vi "Channel Fault - Single.vi"() -> ()   [LabVIEW 2010]
doc: "NI VeriStand custom UI element to fault a single channel. Right-Click on the UI icon to bring up the channel selection dialog and choose a channel. The Path and current value will be displayed.\n\nIn order to fault a channel, set the 'Fault Value' and click the 'Fault Channel?' button. To clear the fault for that channel, click the 'Fault Channel?' button again (so it is false / off)"
uses:
  <vilib>/NI VeriStand/Display Template Support/Display Template Support.llb/cluster_Screen Item Settings.ctl
  <vilib>/NI VeriStand/Display Template Support/Display Template Support.llb/cluster_Graph Scale Settings.ctl
  <vilib>/NI VeriStand/Display Template Support/Display Template Support.llb/cluster_Graph Plot Settings.ctl
  NationalInstruments.VeriStand.SystemStorage
  <vilib>/NI VeriStand/Display Template Support/Display Template Support.llb/enum_Display Template Handler Minimal To Widget Msg.ctl
  <vilib>/NI VeriStand/Display Template Support/Display Template Support.llb/enum_Display Template Handler Minimal To Workspace.ctl
  Data Typedef.ctl
  <vilib>/NI VeriStand/Display Template Support/Display Template Support.llb/sub_Display Template Handler Custom.vi
  <vilib>/NI VeriStand/Execution/Workspace/NI VeriStand - Get Single Channel Value.vi
  <vilib>/NI Veristand/Execution/Workspace/NI_VS Workspace ExecutionAPI.lvlib
  <vilib>/NI Veristand/Execution/ChannelFaultManager/NI_VS ChannelFault ExecutionAPI.lvlib
panel:
  in  "NIVS.System Definition Root":refnum<k24>
  in  "NIVS.Gateway IP Address":string
  out "Fault Channel Full Path":string
  in  "Fault Channel?":bool
  out "Current Value":dbl
  in  "Fault Value":dbl
  in  "Item.Data":T1
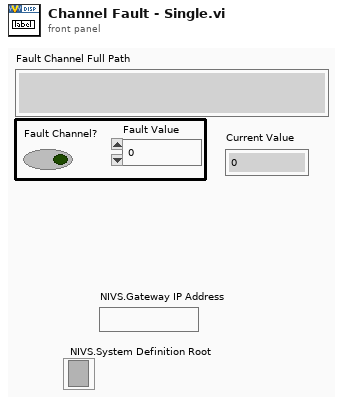
[diagram p1: front panel]
types:
  T1 = typedef "cluster_Screen Item Settings.ctl" = cluster{"Template VI":string, "Position X":i32, "Position Y":i32, "Custom":string, "Show Title Bar":bool, "ID":i32, "Always On Top":bool, "Allow Resize":bool, "Allow Minimize":bool, "Allow Close":bool, "Size to Screen":bool, "Screen.ID":i32, "State":enum16{"Normal", "New"}, "Title":string, "Window Bounds":cluster{"[0]":i16, "[1]":i16, "[2]":i16, "[3]":i16}, "Channel Ref":u64, "Unit":string, "Default Units?":bool, "Flash Limit?":bool, "Color 1":u32, "Color 2":u32, "Color 3":u32, "Color 4":u32, "Bck Color":u32, "Fore Color":u32, "Limit 1":dbl, "Limit 2":dbl, "Limit 3":dbl, "Limit 4":dbl, "Limit Mode 1":i32, "Limit Mode 2":i32, "Limit Mode 3":i32, "Limit Mode 4":i32, "Scale Precision":i32, "Scale Min":dbl, "Scale Max":dbl, "Format":i32, "Precision":i32, "Background Type":i32, "IDs":i32[], "Units":string[], "Labels":string[], "Scale Factor":dbl, "Scale Offset":dbl, "YScale Index":u32[], "XScale":T2, "YScales":T2[], "Plots":T3[], "Update Period":dbl, "History Length":dbl, "My.Ref":refnum<vi>, "Is Control?":bool, "Channel Paths":string[], "Custom Data":variant}
  T2 = typedef "cluster_Graph Scale Settings.ctl" = cluster{"Format":u8, "Precision":u8, "Fit":u8, "Label":string, "Use Default Label":bool, "Label Visible":bool, "Min":dbl, "Max":dbl}
  T3 = typedef "cluster_Graph Plot Settings.ctl" = cluster{"Bar Style":u8, "Fill To":i16, "Fill/PtColor":u32, "Line Style":u8, "Line Width":u8, "Color":u32, "Interp":u8, "Point Style":u8}
  T4 = typedef "enum_Display Template Handler Minimal To Workspace.ctl" = cluster{"Operation":enum16{"SetCustomData", "DeleteItem"}, "Data":variant}
  T5 = typedef "enum_Display Template Handler Minimal To Widget Msg.ctl" = enum16{"Stop", "LaunchConfigDialog"}
  T6 = typedef "Data Typedef.ctl" = cluster{"Fault Channel Full Path":string, "Fault Channel NodePathArray":string[]}
  T7 = typedef "NI_VS Workspace ExecutionAPI.lvlib/WorkspaceAPI.ctl" = refnum<k24>
  T8 = typedef "NI_VS ChannelFault ExecutionAPI.lvlib/ChannelFaultAPI.ctl" = refnum<k24>
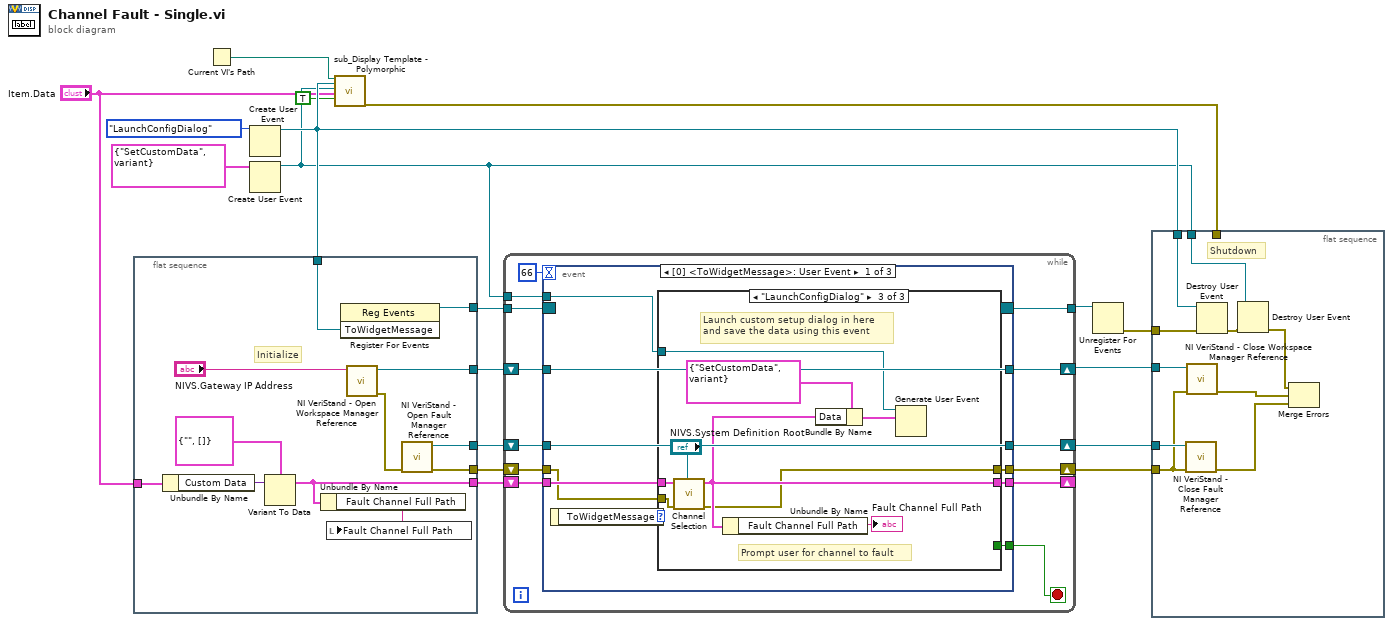
[diagram p0: block diagram]
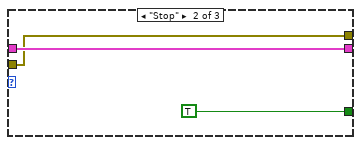
[diagram p3: hidden frame]
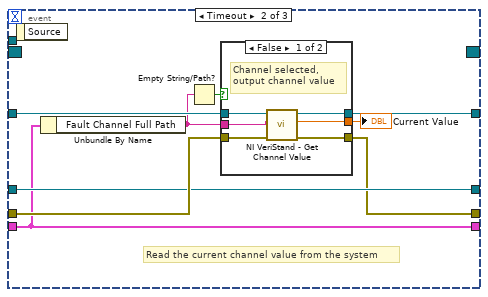
[diagram p4: hidden frame]
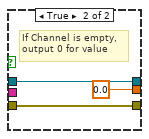
[diagram p5: hidden frame]
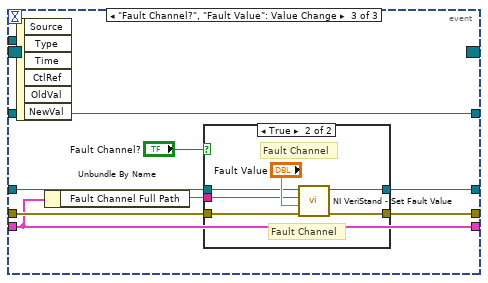
[diagram p6: hidden frame]
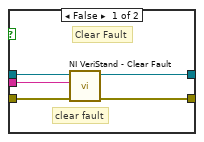
[diagram p7: hidden frame]
diagram:
  n1 = flat-sequence {
    tunnel: [w30] -> w16
    tunnel: w13 -> [w29]
    tunnel: "Item.Data" -> [w28]
    tunnel: [w26] -> w7
    tunnel: [w25] -> w6
    tunnel: [w23] -> w3
    tunnel: [w21] -> w1
    frame #0 {
      # "Initialize"
      n2 = Unbundle By Name(w28) -> ("Custom Data"=w27:variant)
      n3 = Variant To Data(Variant=w27, type=T6 {"Fault Channel Full Path"="", "Fault Channel NodePathArray"=[]}) -> (data=w21:T6)  [unwired: 1 in, 1 out]
      n4 = Unbundle By Name(w21) -> ("Fault Channel Full Path"=w20:string)
      n5 = local write "Fault Channel Full Path"(w20) -> ()
      n6 = register-events(w29) -> (reference out=w30:refnum<event-registration>)  [unwired: 2 in, 1 out]
      n7 = call <vilib>:"NI VeriStand - Open Workspace Manager Reference.vi"("Gateway IP Address (\"\": localhost)"="NIVS.Gateway IP Address") -> ("error out"=w24:errorcluster, "WorkspaceManager"=w26:T7)  [unwired: 9 in]
      n8 = call <vilib>:"NI VeriStand - Open Fault Manager Reference.vi"("error in (no error)"=w24) -> ("error out"=w23:errorcluster, "ChannelFault"=w25:T8)  [unwired: 9 in]
    }
  }
  n9 = Current VI's Path() -> (path=w11:path)
  n10 = Create User Event(user event datatype=enum_Display_Template_Handler_Minimal_To_Widget_Msg."LaunchConfigDialog" ("ToWidgetMessage")) -> (user event=w13:refnum<user-event>)  [unwired: 1 in, 1 out]
  n11 = Create User Event(user event datatype=T4 {"Operation"=enum."SetCustomData", "Data"=variant} ("Data")) -> (user event=w9:refnum<user-event>)  [unwired: 1 in, 1 out]
  n12 = call-poly <vilib>:"sub_Display Template - Polymorphic.vi"("Parent.Path"=w11, "ToWidgetEvent"=w13, "ToWorkspace"=w9, "Item.Data"="Item.Data", "Resizable"=TRUE) -> ("error out"=w18:errorcluster)  [unwired: 1 in, 13 out]
  n13 = while {
    tunnel: w16 -> [w43]
    tunnel: [w41] -> w15
    tunnel: w9 -> [w40]
    shift-right: [w36] -> w5
    shift-left: w7 -> [w37]
    shift-right: [w33] -> w4
    shift-left: w6 -> [w34]
    shift-right: [w32] -> w2
    shift-left: w3 -> [w35]
    shift-right: [w31] -> _
    shift-left: w1 -> [w38]
    stop <- w42 stop-if-true
    n14 = event shown="[0] <ToWidgetMessage>: User Event" {
      selector: w43 -> [_ _ _]
      dyn-events: [_ _ _] -> w41
      timeout: 66 -> [_ _ _]
      tunnel: [w50 _ _] -> w42
      tunnel: w40 -> [w51 _ _]
      tunnel: w38 -> [w49 w69 w85]
      tunnel: w37 -> [w47 w74 w92]
      tunnel: [w47 w73 w92] -> w36
      tunnel: w35 -> [w45 w72 w88]
      tunnel: w34 -> [w46 w71 w91]
      tunnel: [w46 w71 w90] -> w33
      tunnel: [w44 w70 w89] -> w32
      tunnel: [w48 w69 w85] -> w31
      event User Event {
        n15 = event-data() -> ("ToWidgetMessage"=w52:T5)  [unwired: 1 out]
        n16 = case shown="\"LaunchConfigDialog\"" w52 {
          tunnel: [_ TRUE _] -> w50
          tunnel: w51 -> [_ _ w66]
          tunnel: w49 -> [w54 w56 w63]
          tunnel: [w54 w56 w61] -> w48
          tunnel: w45 -> [w53 w55 w59]
          tunnel: [w53 w55 w58] -> w44
          frame Default {
          }
          frame "Stop" {
          }
          frame "LaunchConfigDialog" {
            # "Prompt user for channel to fault"
            # "Launch custom setup dialog in here\nand save the data using this event"
            n17 = call "Channel Selection.vi"("error in (no error)"=w59, "NIVS.System Definition Root"="NIVS.System Definition Root", "Input"=w63) -> ("error out"=w58:errorcluster, "Output"=w61:T6)  [unwired: 7 in]
            n18 = Unbundle By Name(w61) -> ("Fault Channel Full Path"=→"Fault Channel Full Path":string)
            n19 = Bundle By Name(cluster=T4 {"Operation"=enum."SetCustomData", "Data"=variant} ("event data"), "Data"=w61) -> (w64:T4)
            n20 = Generate User Event(user event=w66, event data cluster=w64) -> ()  [unwired: 1 in, 2 out]
          }
        }
      }
      event Timeout {
        # "Read the current channel value from the system"
        n21 = event-data() -> ()  [unwired: 2 out]
        n22 = Unbundle By Name(w69) -> ("Fault Channel Full Path"=w67:string)
        n23 = Empty String/Path?(string/path=w67) -> (empty?=w68:bool)
        n24 = case shown="False" w68 {
          tunnel: [w81 0.0 ("Value")] -> w75
          tunnel: w74 -> [w80 w83]
          tunnel: [w79 w83] -> w73
          tunnel: w72 -> [w78 w84]
          tunnel: [w77 w84] -> w70
          tunnel: w67 -> [w76 _]
          frame False {
            # "Channel selected,\noutput channel value"
            n25 = call-poly <vilib>:"NI VeriStand - Get Channel Value.vi"("error in (no error)"=w78, "Channel"=w76, "WorkspaceManager in"=w80) -> ("error out"=w77:errorcluster, "Value"=w81:dbl, "WorkspaceManager out"=w79:T7)  [unwired: 6 in]
          }
          frame True {
            # "If Channel is empty,\noutput 0 for value"
          }
        }
        "Current Value" <- w75
      }
      event "Fault Channel?", "Fault Value": Value Change {
        n26 = event-data() -> ()  [unwired: 7 out]
        n27 = Unbundle By Name(w85) -> ("Fault Channel Full Path"=w87:string)
        n28 = case shown="True" "Fault Channel?" {
          tunnel: w87 -> [w96 w102]
          tunnel: w91 -> [w97 w101]
          tunnel: [w93 w100] -> w90
          tunnel: w88 -> [w95 w99]
          tunnel: [w94 w98] -> w89
          frame False {
            # "clear fault"
            # "Clear Fault"
            n29 = call <vilib>:"NI VeriStand - Clear Fault.vi"("error in (no error)"=w95, "Channel"=w96, "ChannelFault in"=w97) -> ("error out"=w94:errorcluster, "ChannelFault out"=w93:T8)  [unwired: 7 in]
          }
          frame True {
            # "Fault Channel"
            # "Fault Channel"
            n30 = call <vilib>:"NI VeriStand - Set Fault Value.vi"("error in (no error)"=w99, "Fault Value"="Fault Value", "Channel"=w102, "ChannelFault in"=w101) -> ("error out"=w98:errorcluster, "ChannelFault out"=w100:T8)  [unwired: 6 in]
          }
        }
      }
    }
  }
  n31 = Unregister For Events(event registration refnum=w15) -> (error out=w14:errorcluster)  [unwired: 1 in]
  n32 = flat-sequence {
    tunnel: w18 -> [_]
    tunnel: w14 -> [w112]
    tunnel: w13 -> [w113]
    tunnel: w9 -> [w110]
    tunnel: w5 -> [w109]
    tunnel: w4 -> [w108]
    tunnel: w2 -> [w104]
    frame #0 {
      # "Shutdown"
      n33 = call <vilib>:"NI VeriStand - Close Fault Manager Reference.vi"("error in (no error)"=w104, "ChannelFault"=w108) -> ("error out"=w105:errorcluster)  [unwired: 9 in]
      n34 = call <vilib>:"NI VeriStand - Close Workspace Manager Reference.vi"("error in (no error)"=w104, "WorkspaceManager"=w109) -> ("error out"=w106:errorcluster)  [unwired: 9 in]
      n35 = Destroy User Event(user event=w113, error in=w112) -> (error out=w111:errorcluster)
      n36 = Destroy User Event(user event=w110, error in=w111) -> (error out=w107:errorcluster)
      n37 = Merge Errors(w107, w106, w105) -> ()  [unwired: 1 out]
    }
  }
